vi "FGEN Frequency Sweep.vi"() -> ()   [LabVIEW 2021]
doc: "This example demonstrates frequency sweeping with the 5404.The frequency values (calculated using logarithmic spacing) are pre-computed and stored in an array. The sine wave is then updated with the appropriate frequency either on a timed or user-controlled basis."
uses:
  <instrlib>/niFgen/niFgen.llb/niFgen Waveform Type.ctl
panel:
  in  "Single Step":bool
  in  "Duration (ms)/Step":u32=100
  in  "Stop":bool
  in  "Sweep Trigger Type":u16(ring)=1 items=["Triggered Mode", "Timed Mode"]
  in  "# of Frequency Steps":u32=10
  in  "Stop Frequency":dbl=10000000.0 min=9000.0 max=105000000.0 format="%.2p"
  in  "Amplitude (Vp-p)":dbl=2.0 min=0.0 max=10.0 format="%.2p"
  in  "Start Frequency":dbl=1000000.0 min=9000.0 max=105000000.0 format="%.2p"
  in  "FGEN Resource Name":refnum<k15>
  # "Overview: Demonstrates how to configure an NI PXI-5404 to generate a frequency sweep.\nSoftware Requirements: NI-FGEN\nHardware Requirements: PXI-5404 \nInstructions:\n1. Select the FGEN Resource Name as configured in the Measurement & Automation Explorer.\n2. Specify the Amplitude (Vp-p) that will be used.\n3. Specify the Start Frequency that will be used.\n4. Specify the Stop Frequency that will be used.\n5. Specify the # of Frequency Steps that will be used.\n6. Select the Sweep Trigger Type that will be used.\n7. If you selected Timed Mode for the  Sweep Trigger Type, specify the Duration (ms)/Step.\n8. Run the VI.\n9. If you selected Triggered Mode for the Sweep Trigger Type, click on Single Step to change the frequency to the next frequency step.  \n10. Click Stop to stop the VI."
  # "Triggered"
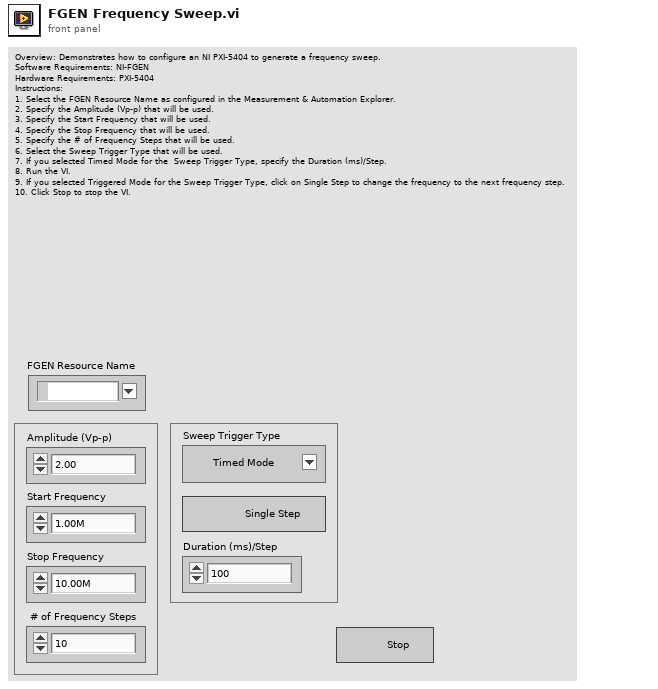
[diagram p1: front panel]
types:
  T1 = typedef "niFgen Waveform Type.ctl" = i32
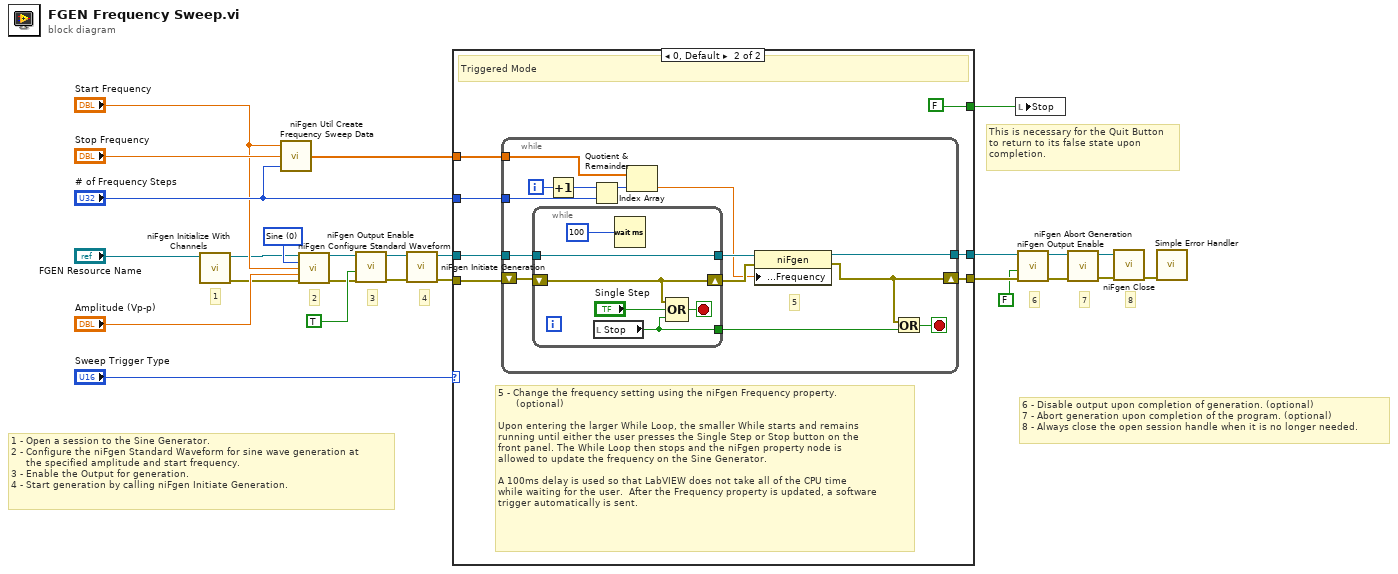
[diagram p0: block diagram]
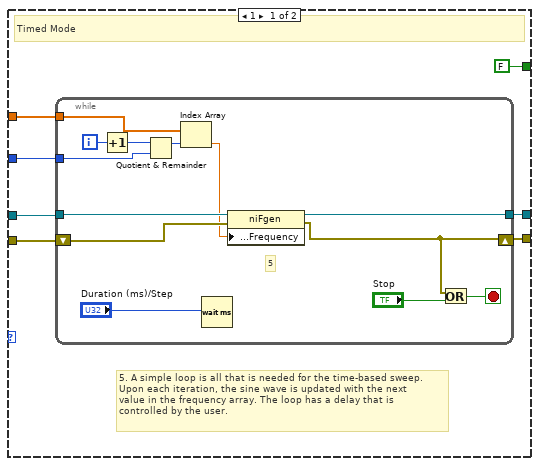
[diagram p2: hidden frame]
diagram:
  w16 = T1 0 items=["Sine", "Square", "Triangle", "Ramp Up", "Ramp Down", "DC", "Noise", "User"] ("waveform")
  # "This is necessary for the Quit Button\nto return to its false state upon\ncompletion."
  # "8"
  # "7"
  # "6"
  # "4"
  # "3"
  # "2"
  # "1"
  # "6 - Disable output upon completion of generation. (optional)\n7 - Abort generation upon completion of the program. (optional)\n8 - Always close the open session handle when it is no longer needed."
  # "1 - Open a session to the Sine Generator.\n2 - Configure the niFgen Standard Waveform for sine wave generation at\n     the specified amplitude and start frequency.\n3 - Enable the Output for generation.\n4 - Start generation by calling niFgen Initiate Generation."
  n1 = call <instrlib>:"niFgen Initialize With Channels.vi"("Resource Name"="FGEN Resource Name") -> ("error out"=w3:errorcluster, "Instrument Handle Out"=w2:refnum<k15>)  [unwired: 9 in]
  n2 = call <instrlib>:"niFgen Util Create Frequency Sweep Data.vi"("# Frequency Steps"="# of Frequency Steps", "Stop Frequency"="Stop Frequency", "Start Frequency"="Start Frequency") -> ("Frequency Sweep Array"=w20:dbl[])
  n3 = call <instrlib>:"niFgen Configure Standard Waveform.vi"("Instrument Handle"=w2, "Waveform"=w16, "Frequency"="Start Frequency", "Amplitude"="Amplitude (Vp-p)", "error in (no error)"=w3) -> ("Instrument Handle Out"=w9:refnum<k15>, "error out"=w10:errorcluster)  [unwired: 9 in]
  n4 = call <instrlib>:"niFgen Output Enable.vi"("error in (no error)"=w10, "Output Enable (default: True)"=TRUE ("output enable"), "Instrument Handle"=w9) -> ("error out"=w21:errorcluster, "Instrument Handle Out"=w8:refnum<k15>)  [unwired: 7 in]
  n5 = call <instrlib>:"niFgen Initiate Generation.vi"("error in (no error)"=w21, "Instrument Handle"=w8) -> ("error out"=w6:errorcluster, "Instrument Handle Out"=w7:refnum<k15>)  [unwired: 8 in]
  n6 = case shown="0, Default" "Sweep Trigger Type" {
    tunnel: w7 -> [w31 w49]
    tunnel: w6 -> [w30 w50]
    tunnel: [w33 w52] -> w26
    tunnel: [w32 w51] -> w25
    tunnel: w20 -> [w29 w48]
    tunnel: "# of Frequency Steps" -> [w28 w47]
    tunnel: [FALSE FALSE] -> w11
    frame 1 {
      # "5. A simple loop is all that is needed for the time-based sweep.\nUpon each iteration, the sine wave is updated with the next\nvalue in the frequency array. The loop has a delay that is\ncontrolled by the user."
      # "Timed Mode"
      n7 = while {
        tunnel: w28 -> [w34]
        tunnel: w29 -> [w40]
        tunnel: [w44] -> w33
        tunnel: w31 -> [w46]
        shift-right: [w35] -> w32
        shift-left: w30 -> [w45]
        i -> [w41]
        stop <- w37 stop-if-true
        # "5"
        n8 = Increment(x=w41) -> (x+1=w43:i32)
        n9 = Quotient & Remainder(x=w43, y=w34) -> (x-y*floor(x/y)=w42:u32)  [unwired: 1 out]
        n10 = Index Array(array=w40, index=w42) -> (element=w39:dbl)
        n11 = Wait (ms)(milliseconds to wait="Duration (ms)/Step") -> ()  [unwired: 1 out]
        n12 = property class="niFgen"(reference=w46, error in=w45, "Standard Function:Standard Function Mode:Frequency"=w39) -> (reference out=w44:refnum<k15>, error out=w35:errorcluster)
        n13 = Or(x=w35, y="Stop") -> (x .or. y?=w37:bool)
      }
    }
    frame 0, Default {
      # "5 - Change the frequency setting using the niFgen Frequency property.\n      (optional)\n\nUpon entering the larger While Loop, the smaller While starts and remains\nrunning until either the user presses the Single Step or Stop button on the\nfront panel. The While Loop then stops and the niFgen property node is\nallowed to update the frequency on the Sine Generator.\n\nA 100ms delay is used so that LabVIEW does not take all of the CPU time\nwhile waiting for the user.  After the Frequency property is updated, a software \ntrigger automatically is sent."
      # "Triggered Mode"
      n14 = while {
        tunnel: w48 -> [w56]
        tunnel: [w65] -> w52
        tunnel: w49 -> [w67]
        tunnel: w47 -> [w57]
        shift-right: [w54] -> w51
        shift-left: w50 -> [w55]
        i -> [w63]
        stop <- w58 stop-if-true
        # "5"
        n15 = while {
          tunnel: [w71] -> w59
          tunnel: [w73] -> w66
          tunnel: w67 -> [w73]
          shift-right: [w69] -> w64
          shift-left: w55 -> [w69]
          stop <- w68 stop-if-true
          n16 = local read "Stop"() -> (w71:bool)
          n17 = Wait (ms)(milliseconds to wait=u32 100 ("millisecond multiple")) -> ()  [unwired: 1 out]
          n18 = Compound Arithmetic op=OR(w69, "Single Step", w71) -> (w68:bool)
        }
        n19 = Increment(x=w63) -> (x+1=w62:i32)
        n20 = Quotient & Remainder(x=w62, y=w57) -> (x-y*floor(x/y)=w61:u32)  [unwired: 1 out]
        n21 = Index Array(array=w56, index=w61) -> (element=w60:dbl)
        n22 = property class="niFgen"(reference=w66, error in=w64, "Standard Function:Standard Function Mode:Frequency"=w60) -> (reference out=w65:refnum<k15>, error out=w54:errorcluster)
        n23 = Or(x=w54, y=w59) -> (x .or. y?=w58:bool)
      }
    }
  }
  n24 = local write "Stop"(w11) -> ()
  n25 = call <instrlib>:"niFgen Output Enable.vi"("error in (no error)"=w25, "Output Enable (default: True)"=FALSE ("output enable"), "Instrument Handle"=w26) -> ("error out"=w17:errorcluster, "Instrument Handle Out"=w18:refnum<k15>)  [unwired: 7 in]
  n26 = call <instrlib>:"niFgen Abort Generation.vi"("error in (no error)"=w17, "Instrument Handle"=w18) -> ("error out"=w23:errorcluster, "Instrument Handle Out"=w24:refnum<k15>)  [unwired: 8 in]
  n27 = call <instrlib>:"niFgen Close.vi"("error in (no error)"=w23, "Instrument Handle"=w24) -> ("error out"=w4:errorcluster)  [unwired: 9 in]
  n28 = call <vilib>:"Simple Error Handler.vi"("error in (no error)"=w4) -> ()  [unwired: 4 in, 5 out]
